vi "PXIe-4139 Initialization VI.vi"(8 "error in (no error)":errorcluster, 10 "Custom XML":string, 11 "Device Item Ref in":T1 format="%.0x") -> (0 "error out":errorcluster, 3 "Device Item Ref out":T1 format="%.0x")   [LabVIEW 2023, in "PXIe-4139 Custom Device.lvlib"]
uses:
  PXIe-4139 Custom Device.lvlib
  <vilib>/NI VeriStand/Custom Device API/Custom Device API.lvlib
  <vilib>/NI VeriStand/Custom Device API/Custom Device Loop Type.ctl
  PXIe-4139 Global Variable.vi
  <vilib>/NI VeriStand/Custom Device API/Custom Device Channel Type.ctl
  <vilib>/NI VeriStand/Custom Device API/Custom Device Channel.ctl
  <vilib>/NI VeriStand/Custom Device API/Custom Device Item Ref.ctl
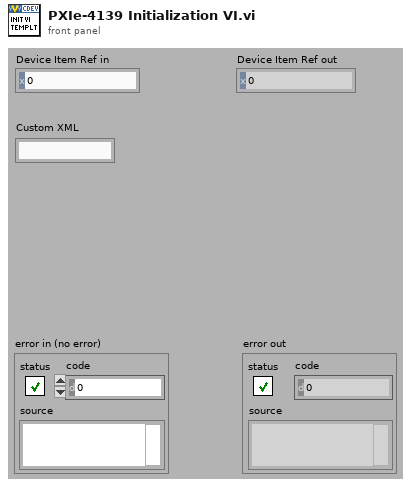
[diagram p1: front panel]
types:
  T1 = typedef "Custom Device API.lvlib/Custom Device Item Ref.ctl" = u64
  T2 = typedef "Custom Device API.lvlib/Custom Device Channel.ctl" = cluster{"Type":T3, "Units":string, "Default Value":dbl, "Faultable":bool, "Scalable":bool}
  T3 = typedef "Custom Device API.lvlib/Custom Device Channel Type.ctl" = enum16{"Input", "Output"}
  T4 = typedef "Custom Device API.lvlib/Custom Device Loop Type.ctl" = enum32{"While Loop", "Timed Loop"}
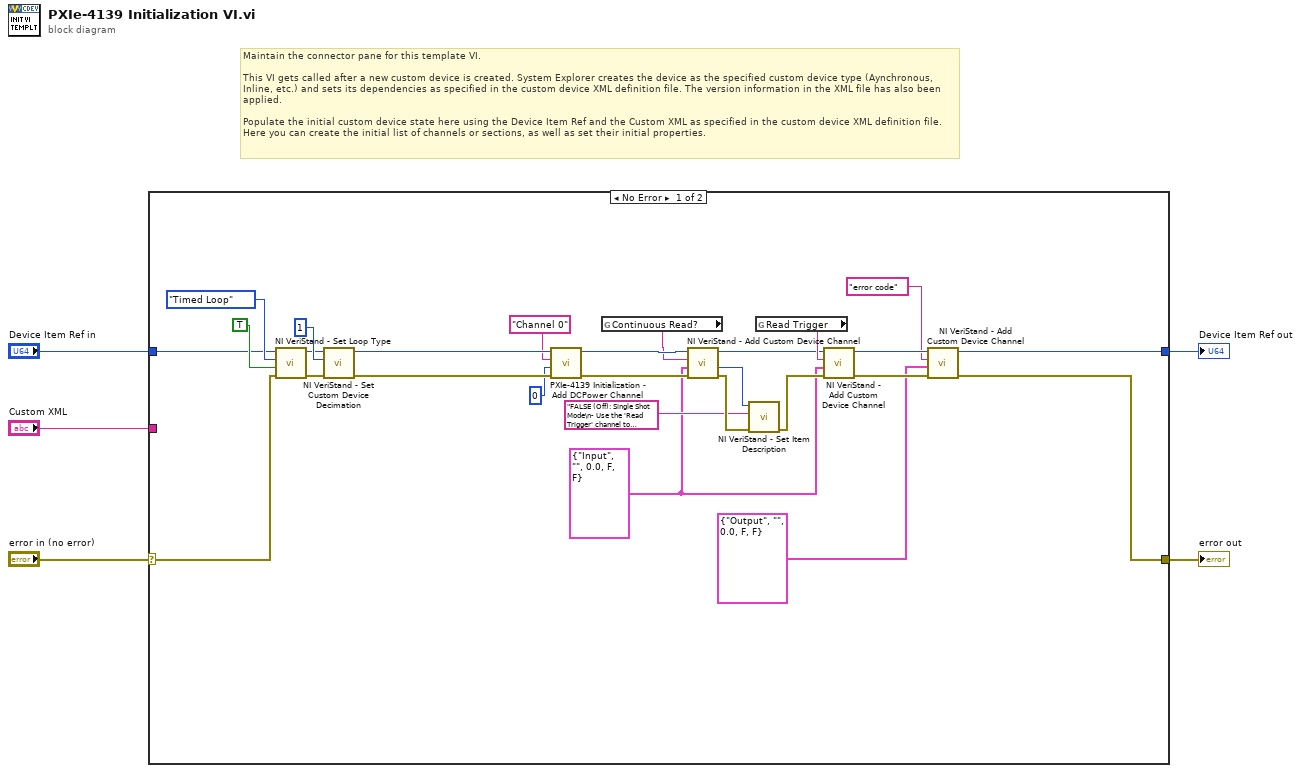
[diagram p0: block diagram]
diagram:
  # "Maintain the connector pane for this template VI.\n\nThis VI gets called after a new custom device is created. System Explorer creates the device as the specified custom device type (Aynchronous, Inline, etc.) and sets its dependencies as specified in the custom device XML definition file. The version information in the XML file has also been applied.\n\nPopulate the initial custom device state here using the Device Item Ref and the Custom XML as specified in the custom device XML definition file. Here you can create the initial list of channels or sections, as well as set their initial properties."
  n1 = case shown="No Error" "error in (no error)" {
    selector: "error in (no error)" -> [w26 w34]
    tunnel: [w7 w34] -> w5
    tunnel: [w8 w33] -> w3
    tunnel: "Device Item Ref in" -> [w27 w33]
    tunnel: "Custom XML" -> [_ _]
    frame No Error {
      w14 = T2 {"Type"=enum."Input", "Units"="", "Default Value"=0.0, "Faultable"=FALSE, "Scalable"=FALSE} ("Channel")
      n2 = call <vilib>:"NI VeriStand - Set Loop Type.vi"("error in (no error)"=w26, "Use Device Clock (Timed Loops only)"=TRUE, "Loop type"=Custom_Device_Loop_Type."Timed Loop", "Device Ref in"=w27) -> ("error out"=w30:errorcluster, "Device Ref out"=w31:T1)  [unwired: 6 in]
      n3 = call <vilib>:"NI VeriStand - Set Custom Device Decimation.vi"("error in (no error)"=w30, "Decimation"=1, "Device Ref in"=w31) -> ("error out"=w25:errorcluster, "Device Ref out"=w24:T1)  [unwired: 7 in]
      n4 = call "PXIe-4139 Initialization - Add DCPower Channel.vi"("error in (no error)"=w25, "Channel #"=0, "Channel Name"="Channel 0", "Device Item Ref In"=w24) -> ("error out"=w21:errorcluster, "Device Item Ref Out"=w22:T1)  [unwired: 6 in]
      n5 = global read "PXIe-4139 Global Variable.vi" "Continuous Read?"() -> (w12:string)
      n6 = call <vilib>:"NI VeriStand - Add Custom Device Channel.vi"("error in (no error)"=w21, "Channel"=w14, "Channel Name"=w12, "Parent Ref in"=w22) -> ("error out"=w17:errorcluster, "Channel Ref"=w18:T1, "Parent Ref out"=w13:T1)  [unwired: 4 in, 1 out]
      n7 = call <vilib>:"NI VeriStand - Set Item Description.vi"("error in (no error)"=w17, "Description"="FALSE (Off): Single Shot Mode\n- Use the 'Read Trigger' channel to execute a single read from the SMU\nTRUE (On): Continuous Read\n- 'Read Trigger' channel is invalid" ("Units"), "Item Ref in"=w18) -> ("error out"=w16:errorcluster)  [unwired: 6 in, 2 out]
      n8 = global read "PXIe-4139 Global Variable.vi" "Read Trigger"() -> (w19:string)
      n9 = call <vilib>:"NI VeriStand - Add Custom Device Channel.vi"("error in (no error)"=w16, "Channel"=w14, "Channel Name"=w19, "Parent Ref in"=w13) -> ("error out"=w11:errorcluster, "Parent Ref out"=w10:T1)  [unwired: 4 in, 2 out]
      n10 = call <vilib>:"NI VeriStand - Add Custom Device Channel.vi"("error in (no error)"=w11, "Channel"=T2 {"Type"=enum."Output", "Units"="", "Default Value"=0.0, "Faultable"=FALSE, "Scalable"=FALSE}, "Channel Name"="error code", "Parent Ref in"=w10) -> ("error out"=w7:errorcluster, "Parent Ref out"=w8:T1)  [unwired: 4 in, 2 out]
    }
    frame Error {
    }
  }
  "error out" <- w5
  "Device Item Ref out" <- w3
